vi "Update.vi"(9 "Column":i32, 10 "Row":i32, 11 "Impenetrable In":refnum<class "Impenetrable.lvclass">) -> (3 "Impenetrable Out":refnum<class "Impenetrable.lvclass">)   [LabVIEW 2015, in "Impenetrable.lvclass"]
uses:
  Impenetrable.lvclass
  Type.ctl
  Common/Position.ctl
  Impenetrable.lvclass/Impenetrable.ctl
  SubVIs/Read-Only Globals.vi
  SubVIs/Globals (private).vi
  Square/Square.lvclass
  Common/Common.lvlib
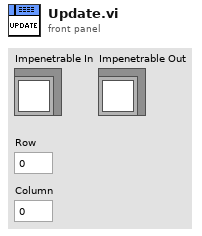
[diagram p1: front panel]
types:
  T1 = typedef "Common.lvlib/Position.ctl" = cluster{"Column":i32, "Row":i32}
  T2 = typedef "Impenetrable.lvclass/Type.ctl" = enum16{"Assassin", "Starter", "Line Starter", "ELine", "WLine", "StartPatrol", "WPatrol", "EPatrol", "WWall", "EWall", "Rain"}
  T3 = typedef "Common.lvlib/Map DVR.ctl" = refnum<data-value>
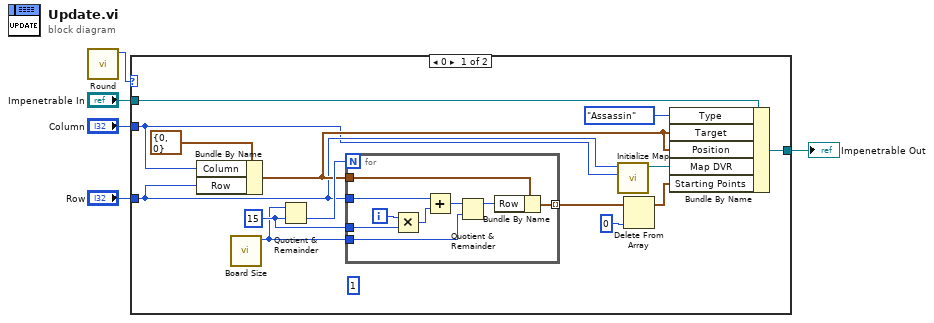
[diagram p0: block diagram]
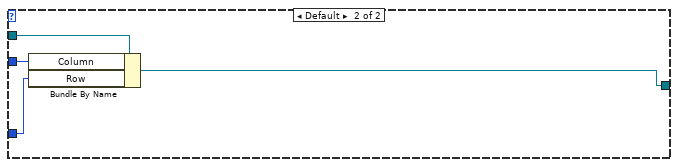
[diagram p2: hidden frame]
diagram:
  n1 = call "Round.vi"() -> ("Round"=w3:i32)  [unwired: 11 in]
  n2 = case shown="0" w3 {
    tunnel: "Impenetrable In" -> [w19 w32]
    tunnel: [w18 w31] -> w4
    tunnel: "Row" -> [w8 w29]
    tunnel: "Column" -> [w7 w30]
    frame 0 {
      w13 = 15 ("y")
      (unwired) 1 ("new element/subarray")
      n3 = Bundle By Name(cluster=T1 {"Column"=0, "Row"=0} ("Center"), "Column"=w7, "Row"=w8) -> (w14:T1)
      n4 = call "Board Size.vi"() -> ("Board Size"=w12:i32)  [unwired: 11 in]
      n5 = Quotient & Remainder(x=w12, y=w13) -> (floor(x/y)=w16:i32)  [unwired: 1 out]
      n6 = for {
        N: w16 -> [_]
        tunnel: w14 -> [w28]
        tunnel: [w27] -> w11 mode=indexing
        tunnel: w8 -> [w26]
        tunnel: w13 -> [w25]
        tunnel: w12 -> [w21]
        i -> [w23]
        n7 = Multiply(x=w23, y=w25) -> (x*y=w24:i32)
        n8 = Add(x=w26, y=w24) -> (x+y=w22:i32)
        n9 = Quotient & Remainder(x=w22, y=w21) -> (x-y*floor(x/y)=w20:i32)  [unwired: 1 out]
        n10 = Bundle By Name(cluster=w28, "Row"=w20) -> (w27:T1)
      }
      n11 = call "Initialize Map.vi"("Column"=w7, "Row"=w8) -> ("Map DVR"=w6:T3)  [unwired: 9 in]
      n12 = Delete From Array(array=w11, index=0) -> (array with subset deleted=w10:T1[])  [unwired: 1 in, 1 out]
      n13 = Bundle By Name(cluster=w19, "Type"=Type."Assassin", "Target"=w14, "Position"=w14, "Map DVR"=w6, "Starting Points"=w10) -> (w18:refnum<class "Impenetrable.lvclass">)
    }
    frame Default {
      n14 = Bundle By Name(cluster=w32, "Column"=w30, "Row"=w29) -> (w31:refnum<class "Impenetrable.lvclass">)
    }
  }
  "Impenetrable Out" <- w4
